vi "Nest Msg Q Multipurpose.vi"(10 "Alias":string, 11 "Actor in":refnum<class "Actor.lvclass">) -> (0 "error out":errorcluster, 1 "Alias found?":bool, 2 "Nest Msg Q":refnum<data-value>, 4 "Alias has duplicate?":bool, 5 "Nest Aliases":string[](array[string]))   [LabVIEW 2021, in "LVCAM.lvlib" / "Actor.lvclass"]
uses:
  Actor.lvclass
  Msg/Msg.lvclass
  Actor.lvclass/Actor.ctl
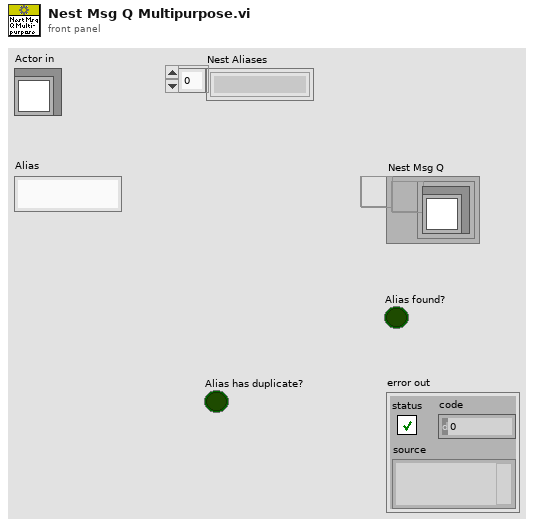
[diagram p1: front panel]
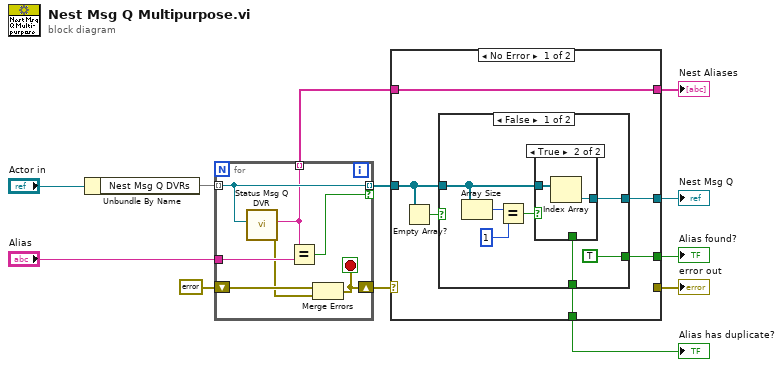
[diagram p0: block diagram]
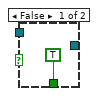
[diagram p2: hidden frame]
diagram:
  n1 = Unbundle By Name("Actor in") -> ("Nest Msg Q DVRs"=w11:set{refnum<data-value>})
  n2 = for {
    tunnel: w11 -> [w15] mode=indexing
    tunnel: [w14] -> w2 mode=indexing
    tunnel: [w15] -> w8 mode=indexing if=w17
    tunnel: "Alias" -> [w18]
    shift-right: [w16] -> w7
    shift-left: errorcluster {"status"=FALSE, "code"=0, "source"=""} ("error out") -> [w19]
    stop <- w16 stop-if-true
    n3 = call "Status Msg Q DVR.vi"("Msg Q DVR"=w15) -> ("error out"=w13:errorcluster, "Msg Q DVR Alias"=w14:string)  [unwired: 9 in]
    n4 = Equal?(x=w14, y=w18) -> (x = y?=w17:bool)
    n5 = Merge Errors(w19, w13) -> (w16:errorcluster)
  }
  n6 = case shown="No Error" w7 {
    selector: w7 -> [_ w36]
    tunnel: w8 -> [w22 _]
    tunnel: [_ w36] -> w6
    tunnel: [w24 _] -> w5
    tunnel: [w23 _] -> w1
    tunnel: [w21 _] -> w4
    tunnel: [w20 _] -> w3
    tunnel: w2 -> [w20 _]
    frame No Error {
      n7 = Empty Array?(array=w22) -> (empty?=w25:bool)
      n8 = case shown="False" w25 {
        tunnel: [TRUE ("Alias found?") _] -> w24
        tunnel: [w29 _] -> w23
        tunnel: w22 -> [w30 _]
        tunnel: [w31 _] -> w21
        frame False {
          n9 = Array Size(array=w30) -> (size(s)=w28:i32)
          n10 = Equal?(x=w28, y=1) -> (x = y?=w26:bool)
          n11 = case shown="True" w26 {
            tunnel: [TRUE ("Alias found?") _] -> w31
            tunnel: w30 -> [_ w35]
            tunnel: [_ w34] -> w29
            frame False {
            }
            frame True {
              n12 = Index Array(array=w35) -> (element=w34:refnum<data-value>)  [unwired: 1 in]
            }
          }
        }
        frame True {
        }
      }
    }
    frame Error {
      # "#LVCAMError"
    }
  }
  "error out" <- w6
  "Nest Aliases" <- w3
  "Alias found?" <- w5
  "Alias has duplicate?" <- w4
  "Nest Msg Q" <- w1
